vi "Read Recipe.vi"(8 "error in (no error)":errorcluster, 11 "Masterv2 in":refnum<class "Masterv2.lvclass">) -> (0 "error out":errorcluster, 3 "Masterv2 out":refnum<class "Masterv2.lvclass">)   [LabVIEW 2014, in "Main Libraryv2.lvlib" / "Masterv2.lvclass"]
uses:
  Master/Masterv2.lvclass
  Stryker/Drying Machine 06.20.2015/CONTROL/Recipes Indicators.ctl
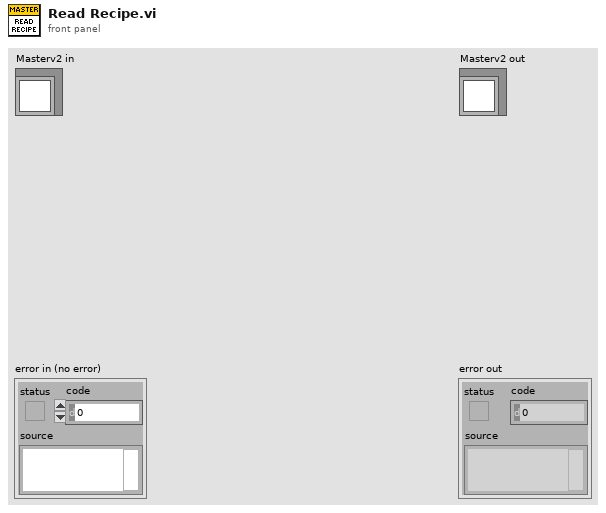
[diagram p1: front panel]
types:
  T1 = typedef "Files Library.lvlib/CONTROL LIBRARY.lvlib/Recipes Indicators.ctl" = cluster{"Speed":string, "Temperature SP":string, "Time Limit":string, "Direction":string}
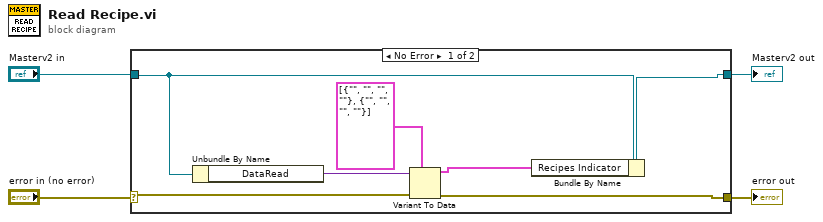
[diagram p0: block diagram]
diagram:
  n1 = case shown="No Error" "error in (no error)" {
    selector: "error in (no error)" -> [w8 w13]
    tunnel: [w7 w13] -> w3
    tunnel: [w5 w12] -> w1
    tunnel: "Masterv2 in" -> [w6 w12]
    frame No Error {
      n2 = Unbundle By Name(w6) -> ("DataRead"=w11:variant)
      n3 = Variant To Data(error in=w8, type=T1[] [{"Speed"="", "Temperature SP"="", "Time Limit"="", "Direction"=""}, {"Speed"="", "Temperature SP"="", "Time Limit"="", "Direction"=""}] ("Recipes Indicator"), Variant=w11) -> (data=w10:T1[], error out=w7:errorcluster)
      n4 = Bundle By Name(cluster=w6, "Recipes Indicator"=w10) -> (w5:refnum<class "Masterv2.lvclass">)
    }
    frame Error {
    }
  }
  "error out" <- w3
  "Masterv2 out" <- w1
